vi "sp_main.vi"() -> ()   [LabVIEW 2009]
panel:
  in  "stop":bool
  out "Digital Inputs":bool[](array[boolean])
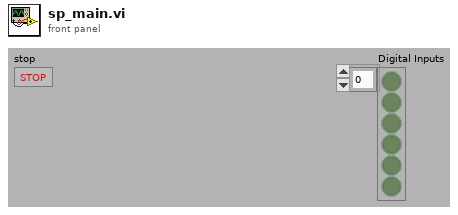
[diagram p1: front panel]
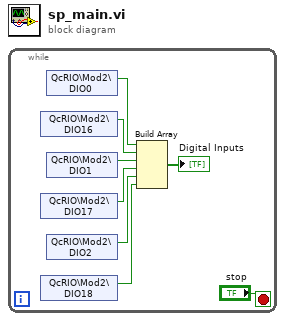
[diagram p0: block diagram]
diagram:
  n1 = while {
    stop <- "stop" stop-if-true
    n2 = shared-variable "QcRIO\\Mod2\\DIO16"() -> (w8:bool)  [unwired: 1 in, 1 out]
    n3 = shared-variable "QcRIO\\Mod2\\DIO17"() -> (w5:bool)  [unwired: 1 in, 1 out]
    n4 = shared-variable "QcRIO\\Mod2\\DIO18"() -> (w3:bool)  [unwired: 1 in, 1 out]
    n5 = shared-variable "QcRIO\\Mod2\\DIO0"() -> (w7:bool)  [unwired: 1 in, 1 out]
    n6 = shared-variable "QcRIO\\Mod2\\DIO1"() -> (w6:bool)  [unwired: 1 in, 1 out]
    n7 = shared-variable "QcRIO\\Mod2\\DIO2"() -> (w4:bool)  [unwired: 1 in, 1 out]
    n8 = Build Array(w7, w8, w6, w5, w4, w3) -> (→"Digital Inputs":bool[])
  }
